vi "Keithley DMM6500 DAQ6500 Series Scanning Temperature.vi"() -> ()   [LabVIEW 2015]
doc: "This example shows how to configure DMM to scanning temperature."
uses:
  <instrlib>/Keithley DMM6500 DAQ6500 Series/Public/Configure/Configure Temperature (Thermocouple).vi
  <instrlib>/Keithley DMM6500 DAQ6500 Series/Public/Data/Read (Multiple Points).vi
  <instrlib>/Keithley DMM6500 DAQ6500 Series/Keithley DMM6500 DAQ6500 Series.lvlib
panel:
  in  "Buffer Element2 ()":i32(ring) items=["", "Date", "Extra", "Formatted", "Fractional", "Reading", "Relative", "Seconds", "Status", "Time", "Tstamp", "Unit", "CHAN", "Extra Form", "Extra Unit"]
  in  "Buffer Element1 ()":i32(ring) items=["", "Date", "Extra", "Formatted", "Fractional", "Reading", "Relative", "Seconds", "Status", "Time", "Tstamp", "Unit", "CHAN", "Extra Format", "Extra Unit"]
  in  "Reference Junction Type (1: Internal)":i32(ring)=1 items=["Simulated", "Internal", "External"]
  in  "Unit (1: Celsius)":i32(ring)=1 items=["Kelvin", "Celsius", "Fahrenheit"]
  in  "Thermocouple Type (3: K)":i32(ring)=3 items=["B", "E", "J", "K", "N", "R", "S", "T"]
  out "Measurements":dbl[](array[numeric])
  in  "Buffer Size (12960)":u32=12960
  in  "Reading Buffer (defbuffer1)":string="defbuffer1"
  in  "Scan Interval (60 s)":dbl=60.0
  in  "Scan Count (1440)":u32=1440
  in  "Channel List (\"2:10\")":string="2:10"
  in  "VISA resource name":refnum<visa-resource-name>
  # "(c) 2018-2022 National Instruments.  ALL RIGHTS RESERVED."
  # "This VI example demonstrates how to use the DMM6500 Series to log temperature measurement data from multiple scan card channels every minute over a 24-hour period using the 2001-TCSCAN card and save that data to an external USB flash drive."
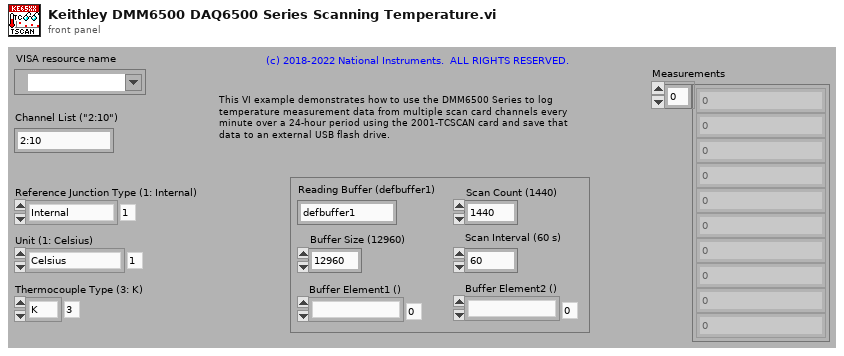
[diagram p1: front panel]
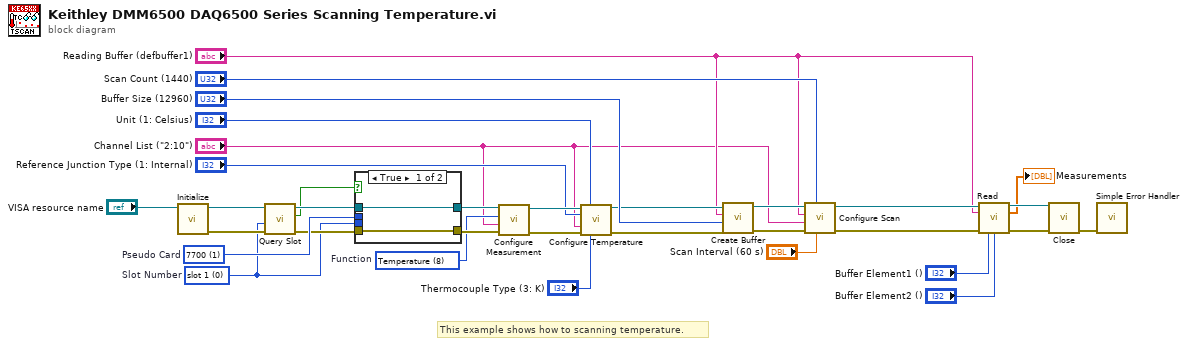
[diagram p0: block diagram]
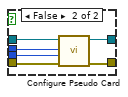
[diagram p2: hidden frame]
diagram:
  w3 = 0 items=["slot 1", "slot 2"]  # Slot Number
  w10 = 1 items=["0", "7700", "7701", "7702", "7703", "7705", "7706", "7707", "7708", "7709", "7710", "7711", "7712"]  # Pseudo Card
  w25 = 8 items=[" Voltage DC", "Voltage AC", "Current DC", "Current AC", "Resistance", "4-wire Resistance", "Diode", "Capacitance", "Temperature", "Continuity", "Frequency", "Period", "Voltage Ratio", "Digitize Voltage", "Digitize Current"]  # Function
  # "This example shows how to scanning temperature."
  n1 = call <instrlib>:"Initialize.vi"("VISA resource name"="VISA resource name") -> ("error out"=w6:errorcluster, "VISA resource name out"=w8:refnum<visa-resource-name>)  [unwired: 9 in]
  n2 = call <instrlib>:"Query Slot.vi"("error in (no error)"=w6, "Slot Number(0: slot 1)"=w3, "VISA resource name"=w8) -> ("error out"=w5:errorcluster, "Real Card In Slot"=w4:bool, "VISA resource name out"=w7:refnum<visa-resource-name>)  [unwired: 6 in]
  n3 = case shown="True" w4 {
    tunnel: [w35 w41] -> w31
    tunnel: [w34 w40] -> w30
    tunnel: w10 -> [_ w39]
    tunnel: w3 -> [_ w38]
    tunnel: w7 -> [w35 w37]
    tunnel: w5 -> [w34 w36]
    frame True {
    }
    frame False {
      n4 = call <instrlib>:"Configure Pseudo Card.vi"("error in (no error)"=w36, "Slot Number (0: slot1)"=w38, "Pseudo Card (0:No pseudocard)"=w39, "VISA resource name"=w37) -> ("error out"=w40:errorcluster, "VISA resource name out"=w41:refnum<visa-resource-name>)  [unwired: 6 in]
    }
  }
  n5 = call <instrlib>:"Configure Measurement.vi"("error in (no error)"=w30, "Channel List(\"\")"="Channel List (\"2:10\")", "Function (0: Voltage DC)"=w25, "VISA resource name"=w31) -> ("error out"=w17:errorcluster, "VISA resource name out"=w18:refnum<visa-resource-name>)  [unwired: 6 in]
  n6 = call-poly <instrlib>:"Configure Temperature.vi"("VISA resource name"=w18, "Unit (1: Celsius)"="Unit (1: Celsius)", "Reference Junction Type (1: Internal)"="Reference Junction Type (1: Internal)", "Channel List(\"\")"="Channel List (\"2:10\")", "error in (no error)"=w17, "Simulated Reference Temperature (0)"="Thermocouple Type (3: K)") -> ("VISA resource name out"=w16:refnum<visa-resource-name>, "error out"=w15:errorcluster)  [unwired: 8 in]
  n7 = call <instrlib>:"Create Buffer.vi"("error in (no error)"=w15, "Buffer Size (10)"="Buffer Size (12960)", "Buffer Name (\"\")"="Reading Buffer (defbuffer1)", "VISA resource name"=w16) -> ("error out"=w26:errorcluster, "VISA resource name out"=w27:refnum<visa-resource-name>)  [unwired: 6 in]
  n8 = call <instrlib>:"Configure Scan.vi"("Delay Seconds (0 s)"="Scan Interval (60 s)", "Scan Count (1)"="Scan Count (1440)", "error in (no error)"=w26, "Channel List(\"\")"="Channel List (\"2:10\")", "Reading Buffer (\"\")"="Reading Buffer (defbuffer1)", "VISA resource name"=w27) -> ("error out"=w21:errorcluster, "VISA resource name out"=w23:refnum<visa-resource-name>)  [unwired: 4 in]
  n9 = call-poly <instrlib>:"Read.vi"("VISA resource name"=w23, "Buffer Name (\"\")"="Reading Buffer (defbuffer1)", "error in (no error)"=w21, "Buffer Element1 ()"="Buffer Element1 ()", "Buffer Element2 ()"="Buffer Element2 ()") -> ("VISA resource name out"=w22:refnum<visa-resource-name>, "Measurements"=→"Measurements":dbl[], "error out"=w20:errorcluster)  [unwired: 8 in]
  n10 = call <instrlib>:"Close.vi"("error in (no error)"=w20, "VISA resource name"=w22) -> ("error out"=w33:errorcluster)  [unwired: 9 in]
  n11 = call <vilib>:"Simple Error Handler.vi"("error in (no error)"=w33) -> ()  [unwired: 4 in, 5 out]
